vi "detectAbsence.vi"(9 "mazeDirection":string, 11 "platforms":i32[](array[numeric])) -> (3 "Boolean":bool)   [LabVIEW 2017]
uses:
  <vilib>/Analysis/baseanly.llb/Mean (DBL).vi
  <vilib>/Analysis/NI_AALBase.lvlib
panel:
  in  "number of consecutive\nmeasurements":i32=5
  # "Channels to weigh"
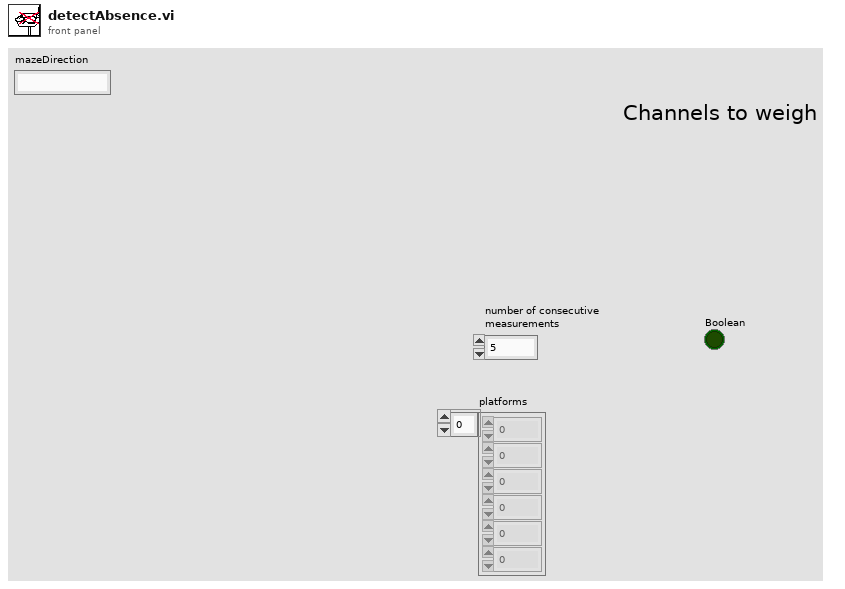
[diagram p1: front panel]
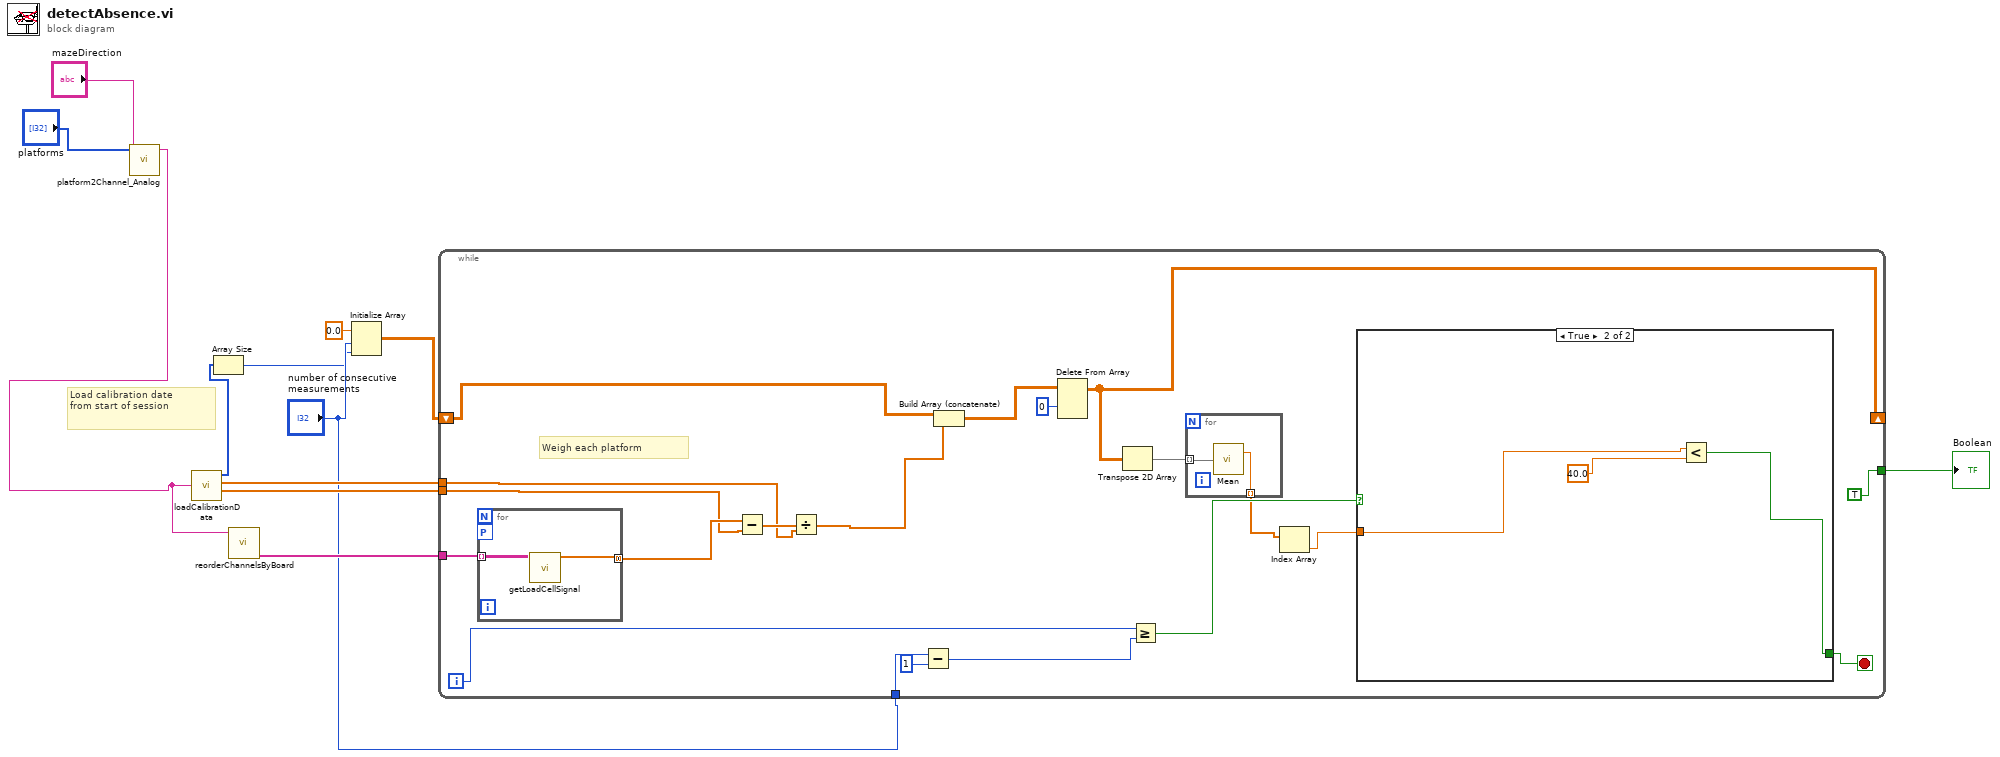
[diagram p0: block diagram]
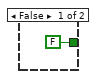
[diagram p2: hidden frame]
diagram:
  # "Load calibration date\nfrom start of session"
  n1 = call "platform2Channel_Analog.vi"("mazeDirection"="mazeDirection", "platforms"="platforms") -> ("DAQmx Channel"=w3:string)  [unwired: 9 in]
  n2 = call "loadCalibrationData.vi"("DAQmx \nPhysical Channel"=w3) -> ("zeroSignals"=w12:dbl[], "voltsPerGram"=w11:dbl[], "index"=w8:i32[])  [unwired: 7 in, 1 out]
  n3 = Array Size(array=w8) -> (size(s)=w5:i32)
  n4 = call "reorderChannelsByBoard.vi"("DAQmx \nPhysical Channel"=w3) -> ("Separated inputs\nas strings"=w10:string[])  [unwired: 8 in, 2 out]
  n5 = Initialize Array(0.0 ("element"), "number of consecutive\nmeasurements", w5) -> (w7:dbl[][])
  n6 = while {
    tunnel: w12 -> [w28]
    tunnel: w11 -> [w31]
    tunnel: w10 -> [w29]
    shift-right: [w20] -> _
    shift-left: w7 -> [w26]
    tunnel: "number of consecutive\nmeasurements" -> [w19]
    tunnel: [TRUE] -> w2
    i -> [w24]
    stop <- w14 stop-if-true
    # "Weigh each platform"
    n7 = for {
      workers-P: _ -> [_]
      tunnel: w29 -> [w40] mode=indexing
      tunnel: [w39] -> w30 mode=concatenating
      n8 = call "getLoadCellSignal.vi"("DAQmx Physical Channel"=w40) -> ("load cell\nsignal"=w39:dbl[])  [unwired: 10 in]
    }
    n9 = Subtract(x=w30, y=w28) -> (x-y=w32:dbl[])
    n10 = Divide(x=w32, y=w31) -> (x/y=w27:dbl[])
    n11 = Subtract(x=w19, y=1) -> (x-y=w17:i32)
    n12 = Build Array (concatenate)(w26, w27) -> (w23:dbl[][])
    n13 = Delete From Array(array=w23, index (row)=0) -> (array with subset deleted=w20:dbl[][])  [unwired: 2 in, 1 out]
    n14 = Transpose 2D Array(2D array=w20) -> (transposed array=w21:dbl[][])
    n15 = Greater Or Equal?(x=w24, y=w17) -> (x >= y?=w25:bool)
    n16 = for {
      tunnel: w21 -> [w34] mode=indexing
      tunnel: [w33] -> w16 mode=indexing
      n17 = call-poly <vilib>:"Mean.vi"("X"=w34) -> ("mean"=w33:dbl)  [unwired: 1 out]
    }
    n18 = Index Array(array=w16) -> (element=w15:dbl)  [unwired: 1 in]
    n19 = case shown="True" w25 {
      tunnel: [FALSE w36] -> w14
      tunnel: w15 -> [_ w37]
      frame False {
      }
      frame True {
        n20 = Less?(x=w37, y=40.0) -> (x < y?=w36:bool)
      }
    }
  }
  "Boolean" <- w2
